vi "auto avance recule.vi"(8 "temps de changement de direction":dbl, 9 "temps":dbl, 10 "vitesse":dbl) -> ()   [LabVIEW 2015]
uses:
  <vilib>/Rock Robotics/WPI/Utilities/WPI_GetSetVariantRefNum.vi
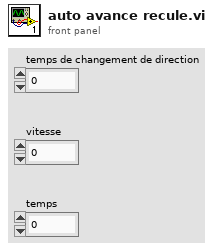
[diagram p1: front panel]
types:
  T1 = typedef "WPI_RobotDriveDevRef.ctl" = cluster{"DevStatus":errorcluster, "Motors[]":T2[], "Square Inputs":bool, "Max Output":dbl}
  T2 = typedef "WPI_MotorControlDeviceRef.ctl" = cluster{"DeviceStatus":errorcluster, "Type":T3, "PWM":cluster{"PWM Channel":T4, "DeadBand":T5}, "CAN":cluster{"Device Number":u8, "Control Mode":T6, "Semaphore":T7, "Max Vout":dbl, "TalonSRX Control Mode":T8}, "Invert":bool}
  T3 = typedef "WPI_MotorControlType.ctl" = enum16{"PWM", "CAN", "CANTalonSRX"}
  T4 = typedef "FPGA_DIOPWMChannel.ctl" = enum8{"PWM 0", "PWM 1", "PWM 2", "PWM 3", "PWM 4", "PWM 5", "PWM 6", "PWM 7", "PWM 8", "PWM 9", "PWM MXP 0", "PWM MXP 1", "PWM MXP 2", "PWM MXP 3", "PWM MXP 4", "PWM MXP 5", "PWM MXP 6", "PWM MXP 7", "PWM MXP 8", "PWM MXP 9", "Invalid"}
  T5 = typedef "WPI_PWMDeadband.ctl" = cluster{"Name":string, "maxPositivePwm":i32, "minPositivePwm":i32, "centerPwm":i32, "maxNegativePwm":i32, "minNegativePwm":i32, "angularRange":u16}
  T6 = typedef "WPI_CANJaguar_ControlMode.ctl" = enum8{"Percent VBus", "Current", "Speed", "Position", "Voltage"}
  T7 = typedef "Semaphore RefNum" = refnum<k1>
  T8 = typedef "WPI_CANTalonSRX_APIControlMode.ctl" = enum8{"Percent VBus", "Speed", "Position", "Slave", "Unchanged / Invalid", "Voltage Compensation", "Current", "Motion Profile"}
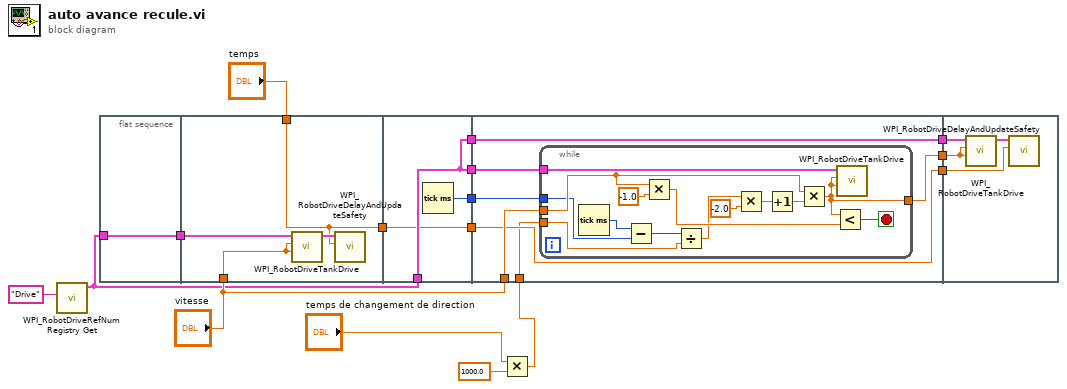
[diagram p0: block diagram]
diagram:
  n1 = call <vilib>:"WPI_RobotDriveRefNum Registry Get.vi"("refnum name"="Drive") -> ("RobotDriveDevRef"=w4:T1)  [unwired: 9 in, 1 out]
  n2 = flat-sequence {
    tunnel: w4 -> [w17]
    tunnel: [w17] -> w16
    tunnel: w16 -> [w20]
    tunnel: "vitesse" -> [w19]
    tunnel: [w18] -> w15
    tunnel: "temps" -> [w18]
    tunnel: [w24] -> w14
    tunnel: [w23] -> w13
    tunnel: w4 -> [w23]
    tunnel: [w23] -> w12
    tunnel: w15 -> [w22]
    tunnel: [w22] -> w11
    tunnel: w14 -> [w31]
    tunnel: w13 -> [w30]
    tunnel: w12 -> [w29]
    tunnel: [w29] -> w10
    tunnel: "vitesse" -> [w28]
    tunnel: [w27] -> w9
    tunnel: w11 -> [w26]
    tunnel: [w26] -> w8
    tunnel: w1 -> [w25]
    tunnel: w10 -> [w48]
    tunnel: w9 -> [w47]
    tunnel: w8 -> [w46]
    frame #0 {
    }
    frame #1 {
      n3 = call <vilib>:"WPI_RobotDriveTankDrive.vi"("Right axis value"=w19, "Left axis value"=w19, "RobotDriveDevRef"=w20) -> ("RobotDriveDevRef"=w21:T1)  [unwired: 6 in, 2 out]
      n4 = call <vilib>:"WPI_RobotDriveDelayAndUpdateSafety.vi"("Delay (s)"=w18, "RobotDriveDevRef"=w21) -> ()  [unwired: 8 in, 2 out]
    }
    frame #2 {
      n5 = Tick Count (ms)() -> (millisecond timer value=w24:u32)
    }
    frame #3 {
      n6 = while {
        tunnel: w31 -> [w39]
        tunnel: w30 -> [w45]
        tunnel: w28 -> [w42]
        tunnel: [w40] -> w27
        tunnel: w25 -> [w37]
        stop <- w44 stop-if-true
        n7 = Tick Count (ms)() -> (millisecond timer value=w38:u32)
        n8 = Subtract(x=w38, y=w39) -> (x-y=w36:u32)
        n9 = Multiply(x=w42, y=-1.0) -> (x*y=w41:dbl)
        n10 = Divide(x=w36, y=w37) -> (x/y=w34:dbl)
        n11 = Multiply(x=w34, y=-2.0) -> (x*y=w33:dbl)
        n12 = Increment(x=w33) -> (x+1=w32:dbl)
        n13 = Multiply(x=w42, y=w32) -> (x*y=w40:dbl)
        n14 = Less?(x=w40, y=w41) -> (x < y?=w44:bool)
        n15 = call <vilib>:"WPI_RobotDriveTankDrive.vi"("Right axis value"=w40, "Left axis value"=w40, "RobotDriveDevRef"=w45) -> ()  [unwired: 6 in, 3 out]
      }
    }
    frame #4 {
      n16 = call <vilib>:"WPI_RobotDriveTankDrive.vi"("Right axis value"=w47, "Left axis value"=w47, "RobotDriveDevRef"=w48) -> ("RobotDriveDevRef"=w49:T1)  [unwired: 6 in, 2 out]
      n17 = call <vilib>:"WPI_RobotDriveDelayAndUpdateSafety.vi"("Delay (s)"=w46, "RobotDriveDevRef"=w49) -> ()  [unwired: 8 in, 2 out]
    }
  }
  n18 = Multiply(x="temps de changement de direction", y=1000.0) -> (x*y=w1:dbl)
